vi "LuaVIEW CIN Spinlock.vi"(0 "action":T2, 1 "refnum in":refnum<vi>, 2 "supplement":string, 5 "LuaVIEW reference in":T3, 7 "index in":i32, 9 "number in":dbl format="%.2f", 11 "string in":string, 12 "boolean in":bool) -> (3 "refnum out":refnum<vi>, 4 "result":T1, 6 "LuaVIEW reference out":T3, 8 "index out":i32, 10 "number out":dbl format="%.2f", 14 "boolean out":bool, 15 "string out":string)   [LabVIEW 2013]
doc: "By calling a subset of LuaVIEW CIN actions through this VI, these actions become protected by a spinlock (since this VI is not reentrant). This is required since these actions manipulate global state (resource tracking list for LuaVIEW states, public function registry, and so on). This VI is private. It should NEVER be used directly by VIs that are not part of the LuaVIEW toolkit."
uses:
  typedefs/t_LuaVIEW CIN Spinlocked Actions.ctl
  typedefs/et_LuaVIEW CIN Results.ctl
  typedefs/t_LuaVIEW Reference.ctl
  typedefs/et_LuaVIEW CIN Actions.ctl
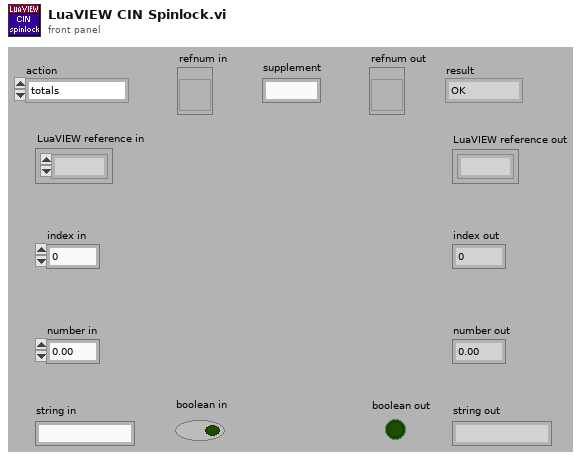
[diagram p1: front panel]
types:
  T1 = typedef "et_LuaVIEW CIN Results.ctl" = enum16{"OK", "error", "main", "call", "clonecall", "modulecall", "exportcall", "index", "yield"}
  T2 = typedef "t_LuaVIEW CIN Spinlocked Actions.ctl" = enum16{"totals", "taskcount", "open", "registerpublic", "registerexport", "revokeexports", "unregnextpublic", "usepublic", "pollexport", "close", "startyieldtest", "endyieldtest", "pollprintbuffer"}
  T3 = typedef "t_LuaVIEW Reference.ctl" = refnum<k1>
  T4 = typedef "et_LuaVIEW CIN Actions.ctl" = enum16{"checksynopsis", "_open", "_registerpublic", "_registerexport", "__never_an_error_result_ns", "luaversion", "cinversion", "_totals", "_taskcount", "pathological", "_unregnextpublic", "registryusecount", "__per_state_actions", "regsetprivate", "regsetindex", "regsetmodule", "_revokeexports", "_usepublic", "prepare", "compile", "execute", "call", "unregstaterefs", "_close", "pullboolean", "pullnumber", "pullI8", "pullU8", "pullI16", "pullU16", "pullI32", "pullU32", "pullobject", "pullrefnum", "pullstring", "pullflat", "pushflat", "pushobject", "getattribute", "setattribute", "stacktostring", "_startyieldtest", "_endyieldtest", "_pollprintbuffer", "__never_an_error_result_ps", "_pollexport", "setclone", "forcecleanup", "gettop", "clearstack", "insert", "pushboolean", "pushnumber", "pushrefnum", "pushstring", "pushnil", "pushvalue", "gettaskref", "settaskref"}
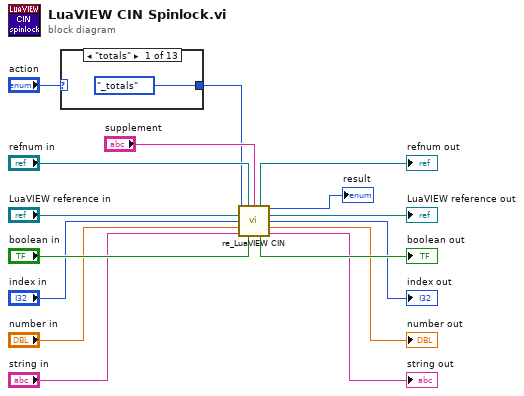
[diagram p0: block diagram]
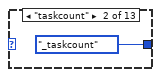
[diagram p2: hidden frame]
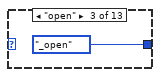
[diagram p3: hidden frame]
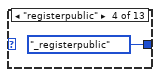
[diagram p4: hidden frame]
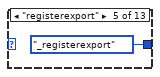
[diagram p5: hidden frame]
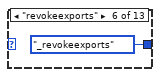
[diagram p6: hidden frame]
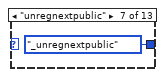
[diagram p7: hidden frame]
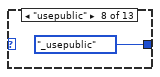
[diagram p8: hidden frame]
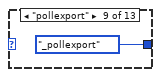
[diagram p9: hidden frame]
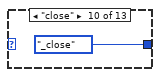
[diagram p10: hidden frame]
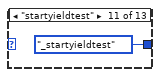
[diagram p11: hidden frame]
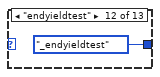
[diagram p12: hidden frame]
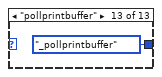
[diagram p13: hidden frame]
diagram:
  n1 = case shown="\"totals\"" "action" {
    tunnel: [et_LuaVIEW_CIN_Actions."_totals" ("action") et_LuaVIEW_CIN_Actions."_taskcount" ("action") et_LuaVIEW_CIN_Actions."_open" ("action") et_LuaVIEW_CIN_Actions."_registerpublic" ("action") et_LuaVIEW_CIN_Actions."_registerexport" ("action") et_LuaVIEW_CIN_Actions."_revokeexports" ("action") et_LuaVIEW_CIN_Actions."_unregnextpublic" ("action") et_LuaVIEW_CIN_Actions."_usepublic" ("action") et_LuaVIEW_CIN_Actions."_pollexport" ("action") et_LuaVIEW_CIN_Actions."_close" ("action") et_LuaVIEW_CIN_Actions."_startyieldtest" ("action") et_LuaVIEW_CIN_Actions."_endyieldtest" ("action") et_LuaVIEW_CIN_Actions."_pollprintbuffer" ("action")] -> w1
    frame "totals" {
    }
    frame "taskcount" {
    }
    frame "open" {
    }
    frame "registerpublic" {
    }
    frame "registerexport" {
    }
    frame "revokeexports" {
    }
    frame "unregnextpublic" {
    }
    frame "usepublic" {
    }
    frame "pollexport" {
    }
    frame "close" {
    }
    frame "startyieldtest" {
    }
    frame "endyieldtest" {
    }
    frame "pollprintbuffer" {
    }
  }
  n2 = call "re_LuaVIEW CIN.vi"("action"=w1, "refnum in"="refnum in", "supplement"="supplement", "LuaVIEW reference in"="LuaVIEW reference in", "index in"="index in", "number in"="number in", "string in"="string in", "boolean in"="boolean in") -> ("refnum out"=→"refnum out":refnum<vi>, "result"=→"result":T1, "LuaVIEW reference out"=→"LuaVIEW reference out":T3, "index out"=→"index out":i32, "number out"=→"number out":dbl, "boolean out"=→"boolean out":bool, "string out"=→"string out":string)  [unwired: 1 in]
